vi "Create Notch Filter (FGV).vi"(6 "fs (Hz)":dbl, 7 "init [F]":bool, 8 "error in (no error)":errorcluster) -> (0 "error out":errorcluster, 2 "IIR Filters":T1(array[cluster]), 5 "init?":bool)   [LabVIEW 2019, in "DSP.lvclass"]
uses:
  DSP.lvclass
panel:
  out "concatenated string":string
  out "harmonics":i32
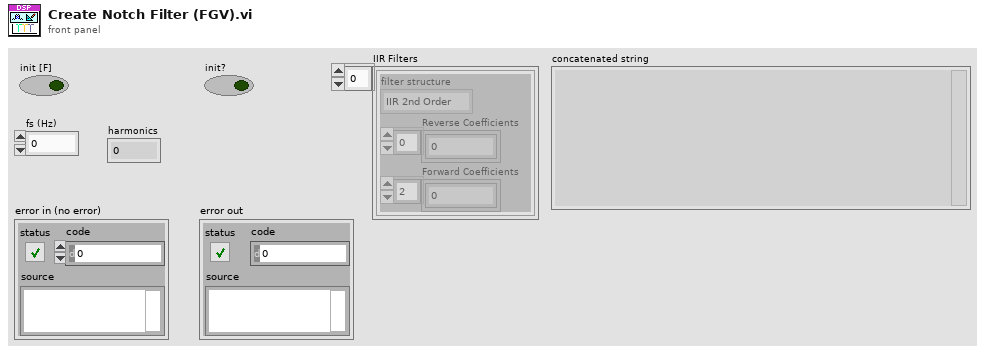
[diagram p1: front panel]
types:
  T1 = cluster{"filter structure":enum32{"IIR 2nd Order", "IIR 4th Order"}, "Reverse Coefficients":dbl[], "Forward Coefficients":dbl[]}[]
  T2 = cluster{"filter structure":enum32{"IIR 2nd Order", "IIR 4th Order"}, "Reverse Coefficients":dbl[], "Forward Coefficients":dbl[]}
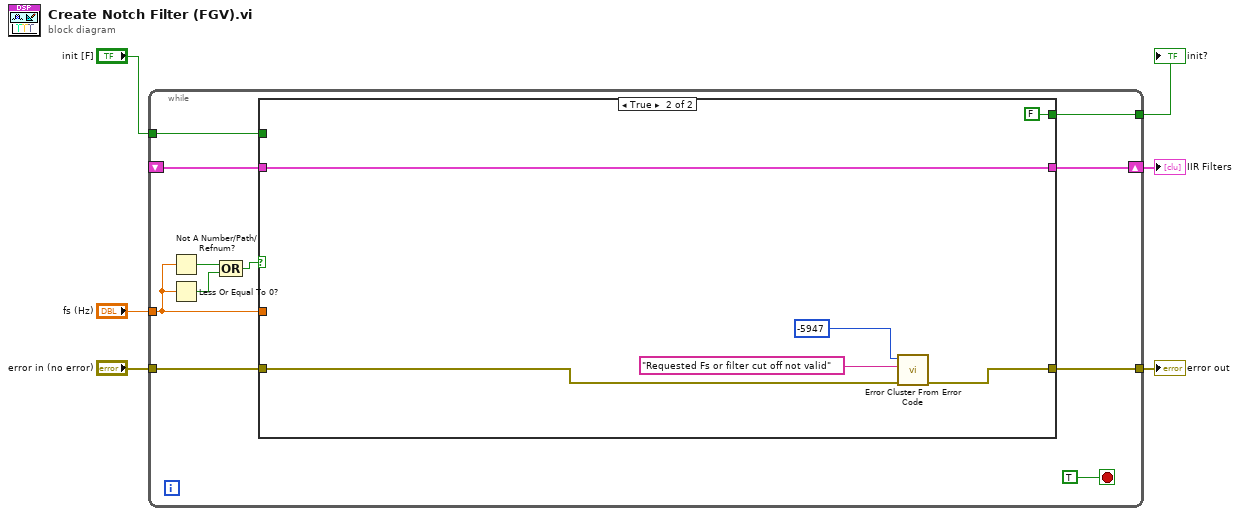
[diagram p0: block diagram]
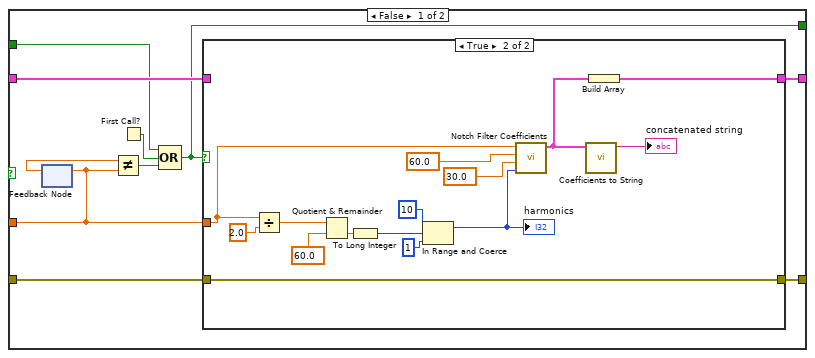
[diagram p2: hidden frame]
diagram:
  n1 = while {
    shift-right: [w16] -> w3
    shift-left: _ -> [w13]
    tunnel: "fs (Hz)" -> [w8]
    tunnel: "error in (no error)" -> [w17]
    tunnel: [w14] -> w6
    tunnel: "init [F]" -> [w11]
    tunnel: [w12] -> w2
    stop <- TRUE stop-if-true
    n2 = Not A Number/Path/Refnum?(number/path/refnum=w8) -> (NaN/Path/Refnum?=w10:bool)
    n3 = Less Or Equal To 0?(x=w8) -> (x <= 0?=w9:bool)
    n4 = Compound Arithmetic op=OR(w10, w9) -> (w7:bool)
    n5 = case shown="True" w7 {
      tunnel: w17 -> [w27 w45]
      tunnel: [w26 w47] -> w16
      tunnel: [w23 w48] -> w14
      tunnel: w13 -> [w22 w47]
      tunnel: w8 -> [w21 _]
      tunnel: [w19 FALSE] -> w12
      tunnel: w11 -> [w18 _]
      frame False {
        n6 = feedback #1() -> (w20:dbl)  [unwired: 1 in]
        n7 = feedback-in #1(w21) -> ()
        n8 = Not Equal?(x=w20, y=w21) -> (x != y?=w25:bool)
        n9 = First Call?() -> (First Call?: T/F=w24:bool)
        n10 = Compound Arithmetic op=OR(w18, w24, w25) -> (w19:bool)
        n11 = case shown="True" w19 {
          tunnel: w27 -> [w28 w44]
          tunnel: [w29 w39] -> w26
          tunnel: w21 -> [_ w30]
          tunnel: [w28 w44] -> w23
          tunnel: w22 -> [w29 _]
          frame False {
          }
          frame True {
            n12 = Divide(x=w30, y=2.0) -> (x/y=w33:dbl)
            n13 = Quotient & Remainder(x=w33, y=60.0 ("f0 [Hz]")) -> (floor(x/y)=w43:dbl)  [unwired: 1 out]
            n14 = To Long Integer(number=w43) -> (32bit integer=w32:i32)
            n15 = In Range and Coerce(upper limit=10, x=w32, lower limit=1) -> (coerced(x)=w36:i32)  [unwired: 1 out]
            "harmonics" <- w36
            n16 = call "Notch Filter Coefficients.vi"("harmonics"=w36, "Q"=30.0 ("Q factor"), "notch (Hz)"=60.0 ("Q factor"), "Sample rate (Hz)"=w30) -> ("IIR Filter Cluster"=w31:T2)  [unwired: 5 in, 2 out]
            n17 = call "Coefficients to String.vi"("IIR Filter Cluster"=w31) -> ("String"=→"concatenated string":string)  [unwired: 10 in]
            n18 = Build Array(w31) -> (w39:T1)
          }
        }
      }
      frame True {
        n19 = call <vilib>:"Error Cluster From Error Code.vi"("error in (no error)"=w45, "error message (\"\")"="Requested Fs or filter cut off not valid" ("error message (\"\")"), "error code (0)"=-5947) -> ("error out"=w48:errorcluster)  [unwired: 6 in]
      }
    }
  }
  "init?" <- w2
  "IIR Filters" <- w3
  "error out" <- w6
